vi "Read UniqueName.vi"(11 "Attribute.Identity in":refnum<class "Attribute.Identity.lvclass">) -> (2 "Unique Name":string, 3 "Attribute.Identity out":refnum<class "Attribute.Identity.lvclass">)   [LabVIEW 2021, in "smo.lvlib" / "Attribute.Identity.lvclass"]
uses:
  Attribute.Identity.lvclass
  Attribute.Identity.lvclass/Attribute.Identity.ctl
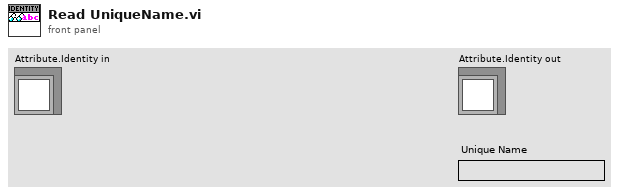
[diagram p1: front panel]
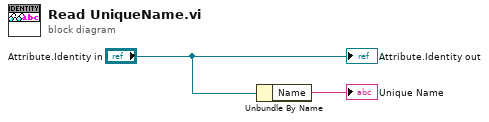
[diagram p0: block diagram]
diagram:
  n1 = Unbundle By Name("Attribute.Identity in") -> ("Name"=→"Unique Name":string)
  "Attribute.Identity out" <- "Attribute.Identity in"
